vi "Initialize Device.vi"(11 "dir":string) -> (2 "function return":u32, 3 "dir out":string)   [LabVIEW 2018, in "Copy of Andor SDK.lvlib"]
doc: "EXPNETTYPE unsigned int WINAPI InitializeDevice(char * dir);"
uses:
  Copy of Andor SDK.lvlib
  <userlib>/Andor SDK/ATMCD32D.dll
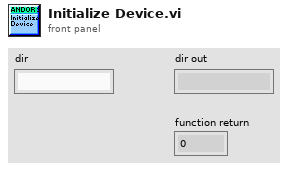
[diagram p1: front panel]
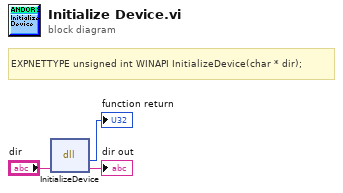
[diagram p0: block diagram]
diagram:
  # "EXPNETTYPE unsigned int WINAPI InitializeDevice(char * dir);"
  n1 = dll-call lib="C:/Program Files (x86)/National Instruments/LabVIEW 2018/user.lib/Andor SDK/ATMCD32D.*" fn="InitializeDevice"("dir"="dir") -> (→"function return":u32, "dir"=→"dir out":string)  [unwired: 3 in, 2 out]
